vi "Clear Error.vi"(7 "error in (no error)":errorcluster) -> (3 "error out":errorcluster)   [LabVIEW 2020, in "RTAF.lvlib"]
uses:
  RTAF.lvlib
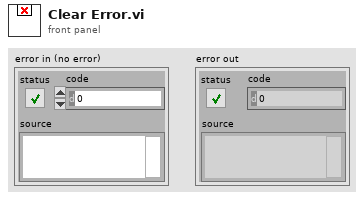
[diagram p1: front panel]
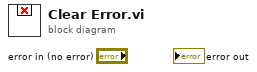
[diagram p0: block diagram]
diagram:
